vi "Drive_Cheezy.vi"(3 "Joystick_In":T1) -> (0 "Right_Motor_Out":dbl, 1 "Left_Motor_Out":dbl)   [LabVIEW 2018]
uses:
  <vilib>/Rock Robotics/WPI/Joystick/WPI_JoystickDevRef.ctl
  <vilib>/Rock Robotics/WPI/Joystick/WPI_JoystickDeviceEnum.ctl
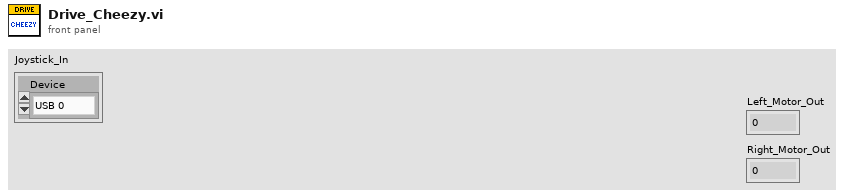
[diagram p1: front panel]
types:
  T1 = typedef "WPI_JoystickDevRef.ctl" = cluster{"Device":T2}
  T2 = typedef "WPI_JoystickDeviceEnum.ctl" = enum16{"USB 0", "USB 1", "USB 2", "USB 3", "USB 4", "USB 5"}
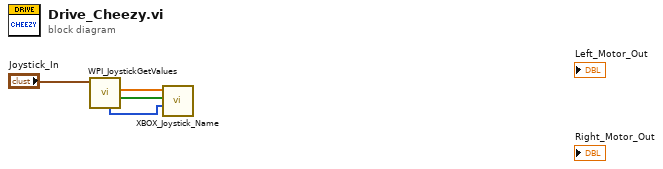
[diagram p0: block diagram]
diagram:
  n1 = call <vilib>:"WPI_JoystickGetValues.vi"("JoystickDevRef"="Joystick_In") -> ("Buttons"=w3:bool[], "Axes"=w4:dbl[], "POVs"=w2:i16[])  [unwired: 6 in, 2 out]
  n2 = call "XBOX_Joystick_Name.vi"("POVs"=w2, "Buttons"=w3, "Axes"=w4) -> ()  [unwired: 7 in, 2 out]
